vi "EAX.vi"(0 "System no.":i32=1 min=1 max=4 step=1, 2 "Axes to command":string[](array[string]), 3 "Enable axis?":bool[](array[boolean]), 5 "error in":errorcluster) -> (19 "error out":errorcluster)   [LabVIEW 2020]
doc: "GCS 3.0\n=====\n\nEAX (Set Axis Activation State)\n\nDescription\nActivates/deactivates the axis by switching its drive on/off.\nMotion of the axis is only possible if the axis is activated with EAX. Activating with EAX passes \nthe axis from the Ready to switch state to the Operation enabled state. For further details, see \n\"Drive State Machine\". \n\nFormat \nEAX <AxisID> <ActivationState>\n\nArguments\n<AxisID>\nAn axis of the controller\nThe available axes can be queried with USG? SYS.\nPossible values: Alias of the axis (p. 94) \n<ActivationState>\nActivation state of the axis\nCorresponds to the switch-on state of the drive of the axis\nPossible values:\n0 = Axis deactivated = Drive switched off\n1 = Axis activated = Drive switched on\n\nResponse\nnone\n\nExample\n>>eax?\n<<AXIS_1=0\n<<AXIS_2=0\n>>eax axis_1 1\n>>eax?\n<<AXIS_1=1\n<<AXIS_2=0\n\nNotes\nIf a motion error occurs, the axis is automatically deactivated on the transition from the Fault \nreaction active state to the Fault state.\nThe activation state of the axes can be queried with the EAX? command. \nThe activation state is also displayed in the status register of the axis, which can be \nqueried with the STV? command. \n\nAttention!\nIf the axis does not have self-locking, deactivating the axis can result in unexpected movements. \nTypical case: In the case of a vertically oriented motion axis, the moving part falls down due to \nits weight force when the drive is switched off.\n-> Take suitable measures to ensure that no unexpected movements are possible when \nthe axis is deactivated.\n\nUser command level\nUSR\n\n\nGCS 2.0\n=====\n\nEnable axis. If disabled, no motion is executed and an error is set. Affected motion sources: motion commands like MOV, MVR, SMO, STE, IMP, SVA, OMA, OMR, MRT, MRW, wave generator commands, macros, analog input, joystick. \nDisabling an axis with EAX stops the axis but does not imply that the motor current is zero. If a motion error occurs axis will be disabled automatically (and servo will be switched off). \nEnabling an axis with EAX will not enable the servo of this axis (SVO.vi). Disabling an axis with EAX will disable the servo status of this axis.\nThe servo status of an axis (SVO.vi) can only be enabled if the axis is enabled (EAX.vi), but enabling the servo with SVO.vi will not change the EAX status of this axis."
panel:
  # "EAX (Set Axis Activation State)\n\nActivates/deactivates the axis by switching its drive on/off.\nMotion of the axis is only possible if the axis is activated with EAX.\nActivating with EAX passes  the axis from the Ready to switch state\nto the Operation enabled state. For further details, see\n\"Drive State Machine\"."
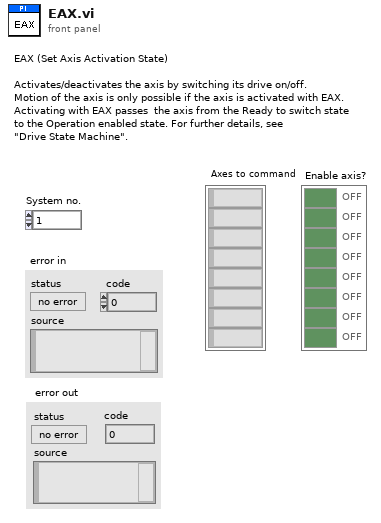
[diagram p1: front panel]
types:
  T1 = typedef "Syntax.ctl" = enum16{"GCS 1.0", "GCS 2.0", "GCS 3.0"}
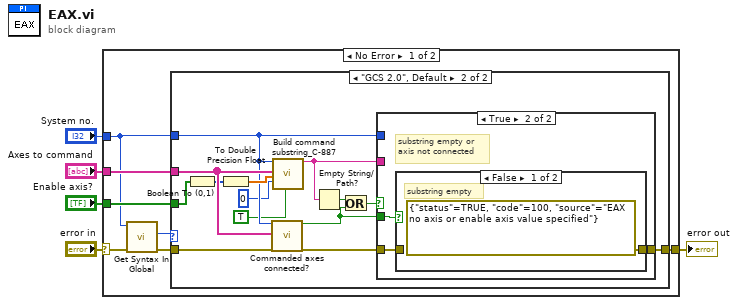
[diagram p0: block diagram]
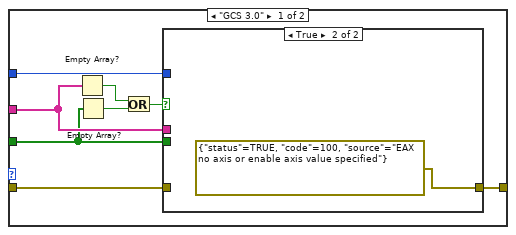
[diagram p2: hidden frame]
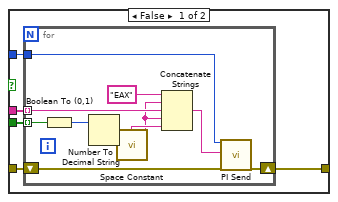
[diagram p3: hidden frame]
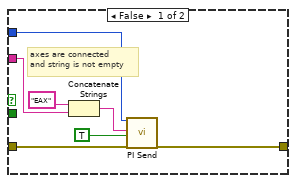
[diagram p4: hidden frame]
diagram:
  n1 = case shown="No Error" "error in" {
    selector: "error in" -> [w9 w63]
    tunnel: [w12 w63] -> w5
    tunnel: "System no." -> [w6 _]
    tunnel: "Axes to command" -> [w11 _]
    tunnel: "Enable axis?" -> [w10 _]
    frame No Error {
      n2 = call "Get Syntax In Global.vi"("error in"=w9, "System no."=w6) -> ("error out"=w8:errorcluster, "Syntax"=w7:T1)  [unwired: 8 in]
      n3 = case shown="\"GCS 2.0\", Default" w7 {
        tunnel: [w20 w50] -> w12
        tunnel: w11 -> [w17 w49]
        tunnel: w10 -> [w14 w47]
        tunnel: w6 -> [w19 w44]
        tunnel: w8 -> [w18 w37]
        frame "GCS 3.0" {
          n4 = Empty Array?(array=w17) -> (empty?=w16:bool)
          n5 = Empty Array?(array=w14) -> (empty?=w13:bool)
          n6 = Or(x=w16, y=w13) -> (x .or. y?=w15:bool)
          n7 = case shown="True" w15 {
            tunnel: w17 -> [w25 _]
            tunnel: w14 -> [w24 _]
            tunnel: [w23 errorcluster {"status"=TRUE, "code"=100, "source"="EAX no axis or enable axis value specified"} ("error out")] -> w20
            tunnel: w19 -> [w22 _]
            tunnel: w18 -> [w21 _]
            frame False {
              n8 = for {
                tunnel: w25 -> [w33] mode=indexing
                tunnel: w24 -> [w35] mode=indexing
                shift-right: [w31] -> w23
                shift-left: w21 -> [w30]
                tunnel: w22 -> [w28]
                n9 = Boolean To (0,1)(Boolean=w35) -> (0, 1=w34:i16)
                n10 = Number To Decimal String(number=w34) -> (decimal integer string=w32:string)  [unwired: 1 in]
                n11 = call <vilib>:"Space Constant.vi"() -> ("String"=w27:string)
                n12 = Concatenate Strings("EAX" ("string"), w27, w33, w27, w32) -> (w29:string)
                n13 = call "PI Send.vi"("System no."=w28, "String to send"=w29, "error in"=w30) -> ("error out"=w31:errorcluster)  [unwired: 3 in, 13 out]
              }
            }
            frame True {
            }
          }
        }
        frame "GCS 2.0", Default {
          n14 = Boolean To (0,1)(Boolean=w47) -> (0, 1=w46:i16[])
          n15 = To Double Precision Float(number=w46) -> (double precision float=w45:dbl[])
          n16 = call "Commanded axes connected?.vi"("System no."=w44, "Commanded axes"=w49, "error in"=w37) -> ("Controller error"=w40:bool, "error out"=w43:errorcluster)  [unwired: 1 in, 14 out]
          n17 = call "Build command substring_C-887.vi"("System no."=w44, "Affected axes"=w49, "Parameters"=w45, "No. of digits"=i16 0 ("No.of digits"), "With space?"=TRUE) -> ("Command substring"=w39:string)  [unwired: 2 in, 12 out]
          n18 = Empty String/Path?(string/path=w39) -> (empty?=w38:bool)
          n19 = Or(x=w38, y=w40) -> (x .or. y?=w48:bool)
          n20 = case shown="True" w48 {
            tunnel: w39 -> [w56 _]
            tunnel: [w52 w60] -> w50
            tunnel: w43 -> [w53 w59]
            tunnel: w44 -> [w51 _]
            tunnel: w40 -> [_ w58]
            frame False {
              # "axes are connected \nand string is not empty"
              n21 = Concatenate Strings("EAX", w56) -> (w54:string)
              n22 = call "PI Send.vi"("System no."=w51, "String to send"=w54, "Attach termination char.?"=TRUE ("Attach Linefeed?"), "error in"=w53) -> ("error out"=w52:errorcluster)  [unwired: 2 in, 13 out]
            }
            frame True {
              # "substring empty or\naxis not connected"
              n23 = case shown="False" w58 {
                tunnel: [errorcluster {"status"=TRUE, "code"=100, "source"="EAX no axis or enable axis value specified"} ("error out") w62] -> w60
                tunnel: w59 -> [_ w62]
                frame False {
                  # "substring empty"
                }
                frame True {
                  # "commanded axis\nnot connected"
                }
              }
            }
          }
        }
      }
    }
    frame Error {
    }
  }
  "error out" <- w5
